vi "NEW_SHIFT_CAL_new.vi"() -> ()   [LabVIEW 2017]
uses:
  <vilib>/addons/database/Connection.llb/DB Tools Open Connec (Path).vi
  <vilib>/addons/database/NI_Database_API.lvlib
panel:
  in  "Cancel Button - Archive":bool
  out "ACTUAL_WORK_TIME":i32
  out "BREAK":i32
  out "LUNCH TIME":i32
  out "In Minutes":i32
  out "error out":errorcluster
  in  "Cycle Time":dbl
  out "x-y":dbl
  out "x-y 8":dbl
  out "x-y 7":dbl
  in  "INCLUDED 9":bool=TRUE
  in  "INCLUDED 8":bool=TRUE
  in  "INCLUDED 7":bool=TRUE
  in  "INCLUDED 6":bool=TRUE
  in  "INCLUDED 5":bool=TRUE
  in  "INCLUDED 4":bool=TRUE
  in  "INCLUDED 3":bool=TRUE
  in  "Include 2":bool=TRUE
  in  "Include":bool=TRUE
  in  "EXTRA SHIFT INCLUDED":bool=TRUE
  in  "Save Button":bool
  in  "Cluster 12":T1 {"1Start 4" format="%<%H:%M:%S>T"; "1Start 3" format="%<%H:%M:%S>T"; "1Start 2" format="%<%H:%M:%S>T"; "1Start" format="%<%H:%M:%S>T"}
  in  "Cluster 11":T1 {"1Start 4" format="%<%H:%M:%S>T"; "1Start 3" format="%<%H:%M:%S>T"; "1Start 2" format="%<%H:%M:%S>T"; "1Start" format="%<%H:%M:%S>T"}
  in  "Cluster 10":T1 {"1Start 4" format="%<%H:%M:%S>T"; "1Start 3" format="%<%H:%M:%S>T"; "1Start 2" format="%<%H:%M:%S>T"; "1Start" format="%<%H:%M:%S>T"}
  in  "Cluster 9":T1 {"1Start 4" format="%<%H:%M:%S>T"; "1Start 3" format="%<%H:%M:%S>T"; "1Start 2" format="%<%H:%M:%S>T"; "1Start" format="%<%H:%M:%S>T"}
  in  "Cluster 8":T2 {"1Start 8" format="%<%H:%M:%S>T"; "1Start 7" format="%<%H:%M:%S>T"; "1Start 6" format="%<%H:%M:%S>T"; "1Start 5" format="%<%H:%M:%S>T"; "1Start 4" format="%<%H:%M:%S>T"; "1Start 3" format="%<%H:%M:%S>T"; "1Start 2" format="%<%H:%M:%S>T"; "1Start" format="%<%H:%M:%S>T"}
  in  "Cluster 7":T2 {"1Start 8" format="%<%H:%M:%S>T"; "1Start 7" format="%<%H:%M:%S>T"; "1Start 6" format="%<%H:%M:%S>T"; "1Start 5" format="%<%H:%M:%S>T"; "1Start 4" format="%<%H:%M:%S>T"; "1Start 3" format="%<%H:%M:%S>T"; "1Start 2" format="%<%H:%M:%S>T"; "1Start" format="%<%H:%M:%S>T"}
  in  "Cluster 6":T2 {"1Start 8" format="%<%H:%M:%S>T"; "1Start 7" format="%<%H:%M:%S>T"; "1Start 6" format="%<%H:%M:%S>T"; "1Start 5" format="%<%H:%M:%S>T"; "1Start 4" format="%<%H:%M:%S>T"; "1Start 3" format="%<%H:%M:%S>T"; "1Start 2" format="%<%H:%M:%S>T"; "1Start" format="%<%H:%M:%S>T"}
  in  "Cluster 5":T2 {"1Start 8" format="%<%H:%M:%S>T"; "1Start 7" format="%<%H:%M:%S>T"; "1Start 6" format="%<%H:%M:%S>T"; "1Start 5" format="%<%H:%M:%S>T"; "1Start 4" format="%<%H:%M:%S>T"; "1Start 3" format="%<%H:%M:%S>T"; "1Start 2" format="%<%H:%M:%S>T"; "1Start" format="%<%H:%M:%S>T"}
  in  "Blank Button":bool
  in  "Cluster 4":T3 {"1Start 6" format="%<%H:%M:%S>T"; "1Start 5" format="%<%H:%M:%S>T"; "1Start 4" format="%<%H:%M:%S>T"; "1Start 3" format="%<%H:%M:%S>T"; "1Start 2" format="%<%H:%M:%S>T"; "1Start" format="%<%H:%M:%S>T"}
  in  "Cluster 3":T3 {"1Start 6" format="%<%I:%M:%S %p>T"; "1Start 5" format="%<%I:%M:%S %p>T"; "1Start 4" format="%<%I:%M:%S %p>T"; "1Start 3" format="%<%I:%M:%S %p>T"; "1Start 2" format="%<%I:%M:%S %p>T"; "1Start" format="%<%I:%M:%S %p>T"}
  in  "Cluster 2":T3 {"1Start 2" format="%<%I:%M:%S %p>T"; "1Start" format="%<%I:%M:%S %p>T"; "1Start 6" format="%<%I:%M:%S %p>T"; "1Start 5" format="%<%I:%M:%S %p>T"; "1Start 4" format="%<%I:%M:%S %p>T"; "1Start 3" format="%<%I:%M:%S %p>T"}
  in  "Cluster":T3 {"1Start 6" format="%<%I:%M:%S %p>T"; "1Start 5" format="%<%I:%M:%S %p>T"; "1Start 4" format="%<%I:%M:%S %p>T"; "1Start 3" format="%<%I:%M:%S %p>T"; "1Start 2" format="%<%I:%M:%S %p>T"; "1Start" format="%<%I:%M:%S %p>T"}
  # "SHIFT SETTING"
  # "06:00:00"
  # "17:59:59"
  # "Sec"
  # "EXTRA SHIFT"
  # "X"
  # "Y"
  # "A"
  # "B"
  # "C"
  # "D"
  # "BREAK 3"
  # "START"
  # "END"
  # "LUNCH"
  # "START"
  # "END"
  # "BREAK 1"
  # "START"
  # "END"
  # "SHIFT IN DAY"
  # "CODE"
  # "START"
  # "END"
  # "A"
  # "B"
  # "C"
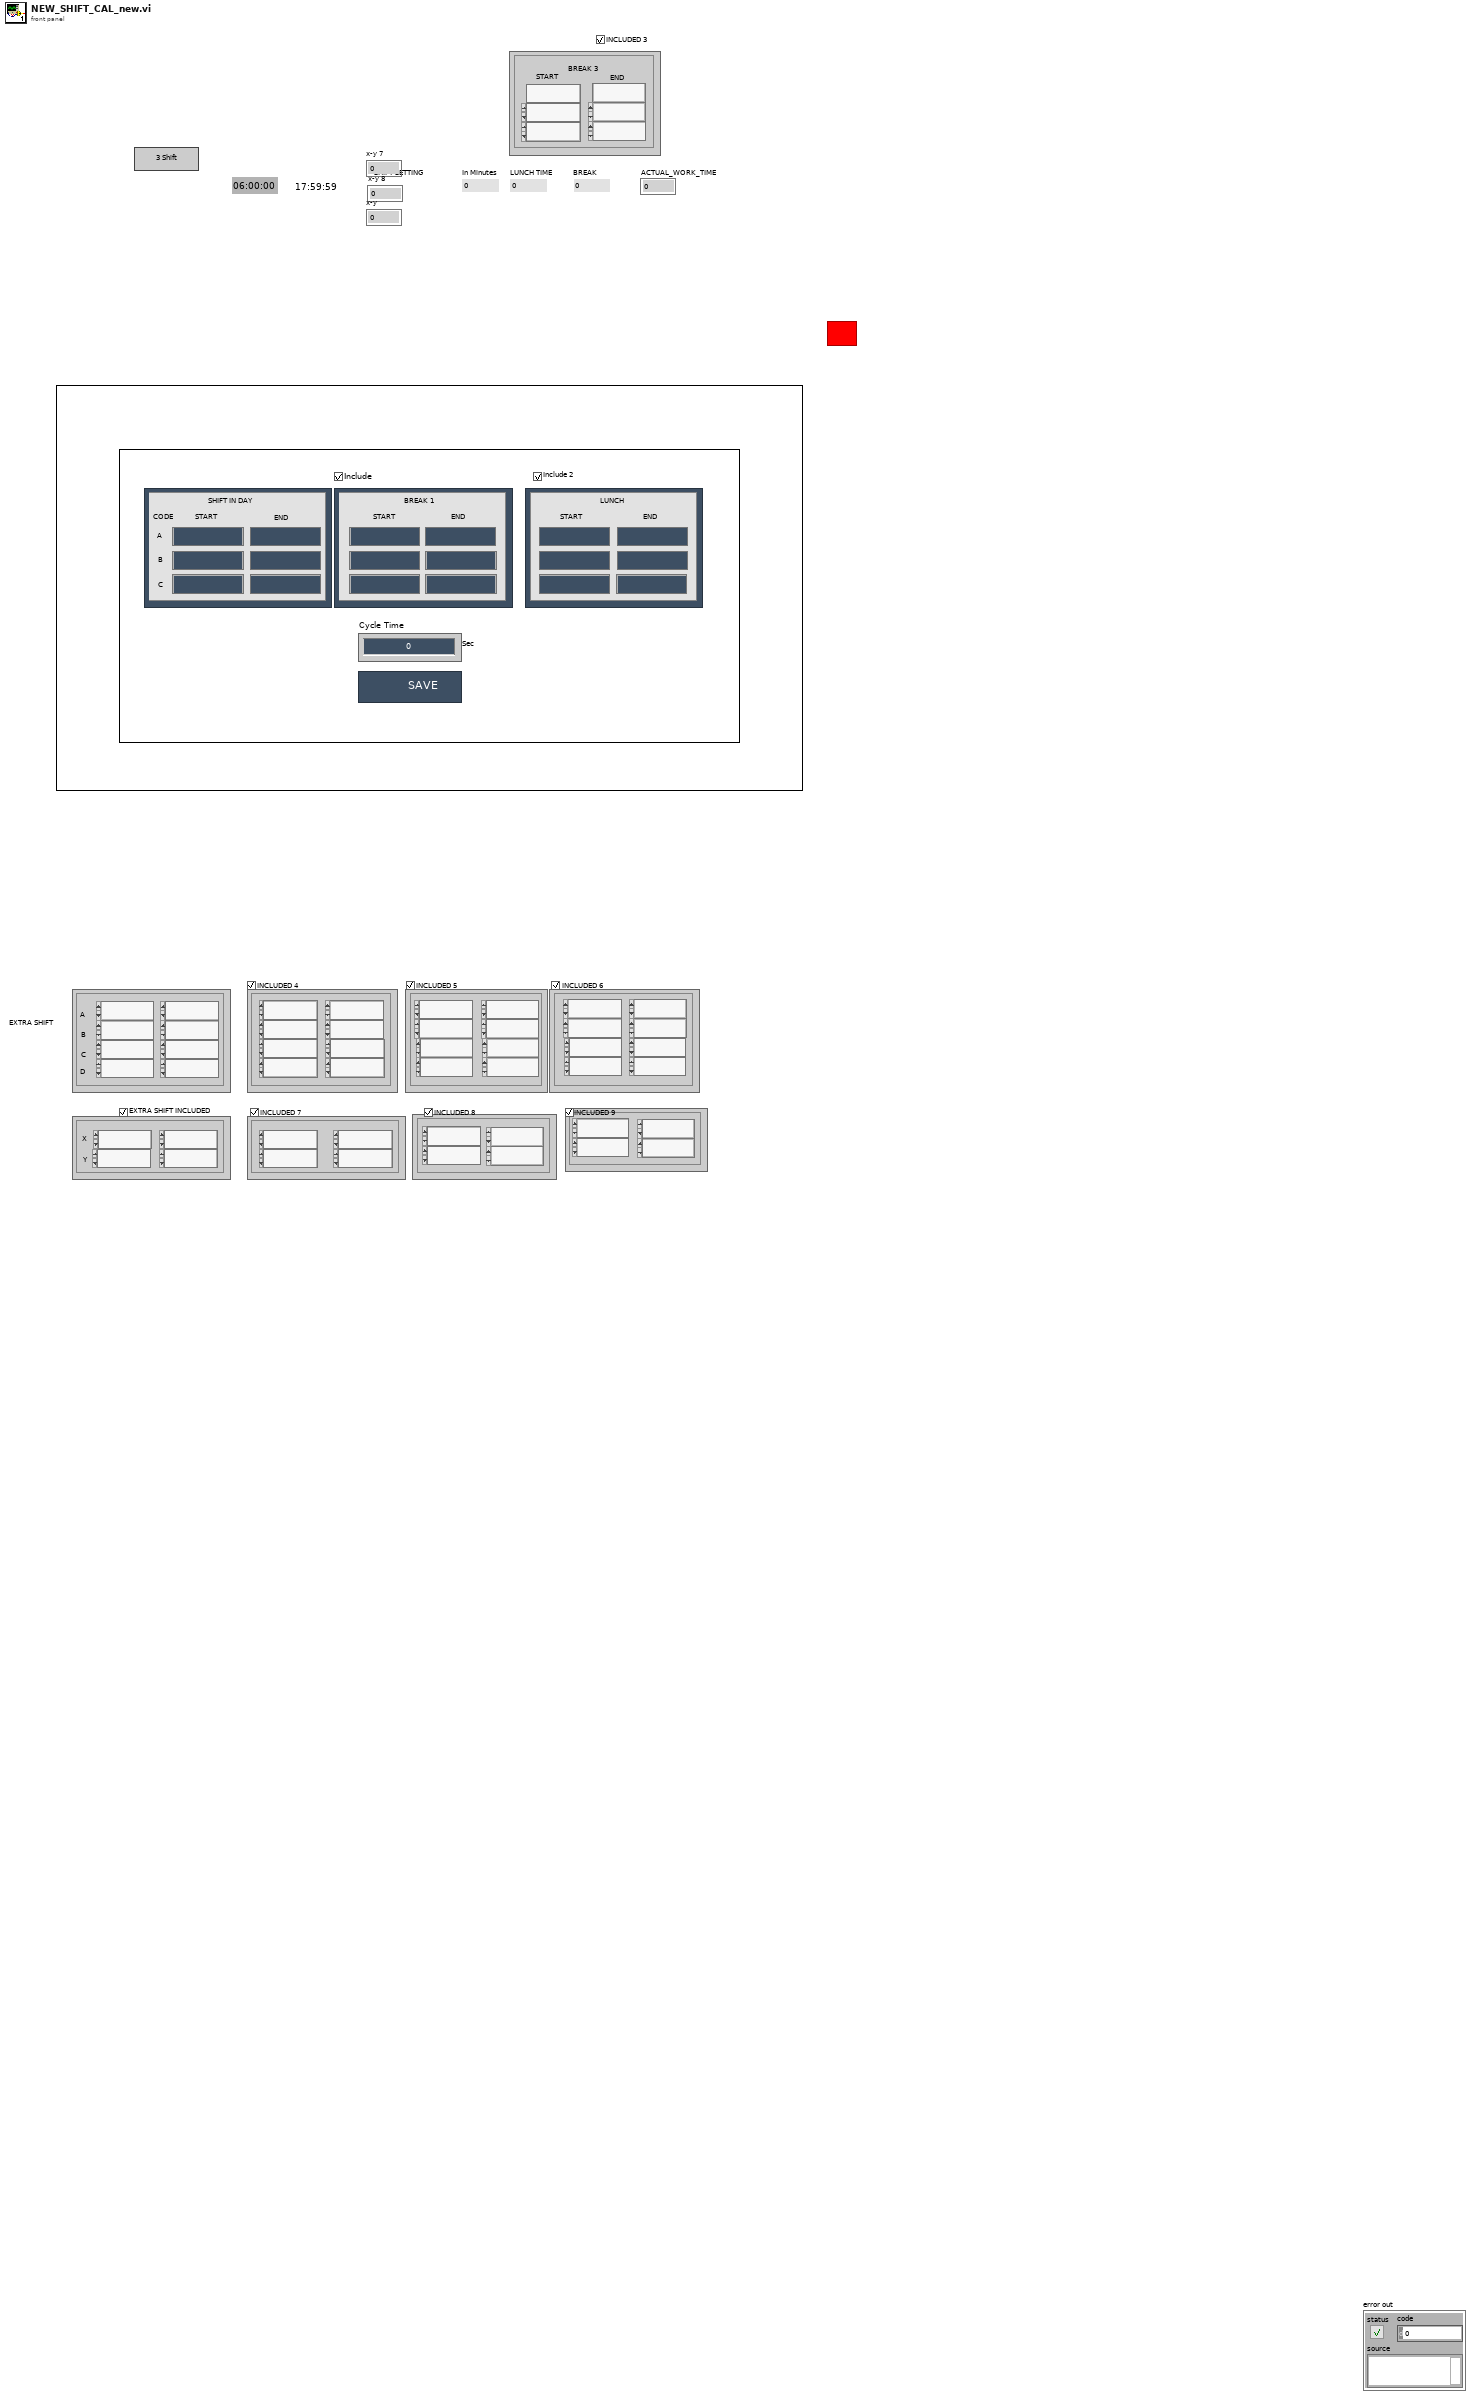
[diagram p1: front panel]
types:
  T1 = cluster{"1Start":timestamp, "1Start 2":timestamp, "1Start 3":timestamp, "1Start 4":timestamp}
  T2 = cluster{"1Start":timestamp, "1Start 2":timestamp, "1Start 3":timestamp, "1Start 4":timestamp, "1Start 5":timestamp, "1Start 6":timestamp, "1Start 7":timestamp, "1Start 8":timestamp}
  T3 = cluster{"1Start":timestamp, "1Start 2":timestamp, "1Start 3":timestamp, "1Start 4":timestamp, "1Start 5":timestamp, "1Start 6":timestamp}
  T4 = typedef "NI_Database_API.lvlib/Conn ObjectReference.ctl" = refnum<k1>
  T5 = cluster{"Time Stamp Out[0]":timestamp, "Time Stamp Out[1]":timestamp, "Time Stamp Out[2]":timestamp, "Time Stamp Out[3]":timestamp}
  T6 = cluster{"Time Stamp Out[0]":timestamp, "Time Stamp Out[1]":timestamp, "Time Stamp Out[2]":timestamp, "Time Stamp Out[3]":timestamp, "Time Stamp Out[4]":timestamp, "Time Stamp Out[5]":timestamp}
  T7 = cluster{"Time Stamp Out[0]":timestamp, "Time Stamp Out[1]":timestamp, "Time Stamp Out[2]":timestamp, "Time Stamp Out[3]":timestamp, "Time Stamp Out[4]":timestamp, "Time Stamp Out[5]":timestamp, "Time Stamp Out[6]":timestamp, "Time Stamp Out[7]":timestamp}
  T8 = cluster{"INCLUDED 9":bool, "date/time string":string, "date/time string":string, "date/time string":string, "date/time string":string}
  T9 = cluster{"INCLUDED 7":bool, "date/time string":string, "date/time string":string, "date/time string":string, "date/time string":string}
  T10 = cluster{"EXTRA SHIFT INCLUDED":bool, "date/time string":string, "date/time string":string, "date/time string":string, "date/time string":string}
  T11 = cluster{"INCLUDED 8":bool, "date/time string":string, "date/time string":string, "date/time string":string, "date/time string":string}
  T12 = cluster{"Include":bool, "date/time string":string, "date/time string":string, "date/time string":string, "date/time string":string, "date/time string":string, "date/time string":string, "In Minutes":i32}
  T13 = cluster{"INCLUDED 4":bool, "date/time string":string, "date/time string":string, "date/time string":string, "date/time string":string, "date/time string":string, "date/time string":string, "date/time string":string, "date/time string":string}
  T14 = cluster{"date/time string":string, "date/time string":string, "date/time string":string, "date/time string":string, "date/time string":string, "date/time string":string, "date/time string":string, "date/time string":string}
  T15 = cluster{"INCLUDED 6":bool, "date/time string":string, "date/time string":string, "date/time string":string, "date/time string":string, "date/time string":string, "date/time string":string, "date/time string":string, "date/time string":string}
  T16 = cluster{"INCLUDED 5":bool, "date/time string":string, "date/time string":string, "date/time string":string, "date/time string":string, "date/time string":string, "date/time string":string, "date/time string":string, "date/time string":string}
  T17 = cluster{"Include 2":bool, "date/time string":string, "date/time string":string, "date/time string":string, "date/time string":string, "date/time string":string, "date/time string":string, "In Minutes":i32}
  T18 = cluster{"INCLUDED 3":bool, "date/time string":string, "date/time string":string, "date/time string":string, "date/time string":string, "date/time string":string, "date/time string":string}
  T19 = cluster{"Blank Button":bool, "date/time string":string, "date/time string":string, "date/time string":string, "date/time string":string, "date/time string":string, "date/time string":string, "In Minutes":i32, i32}
  T20 = cluster{"Time":string, "Time":string, "In Minutes":i32}
  T21 = cluster{"Time":string, "Time":string, "In Minutes":i32}[]
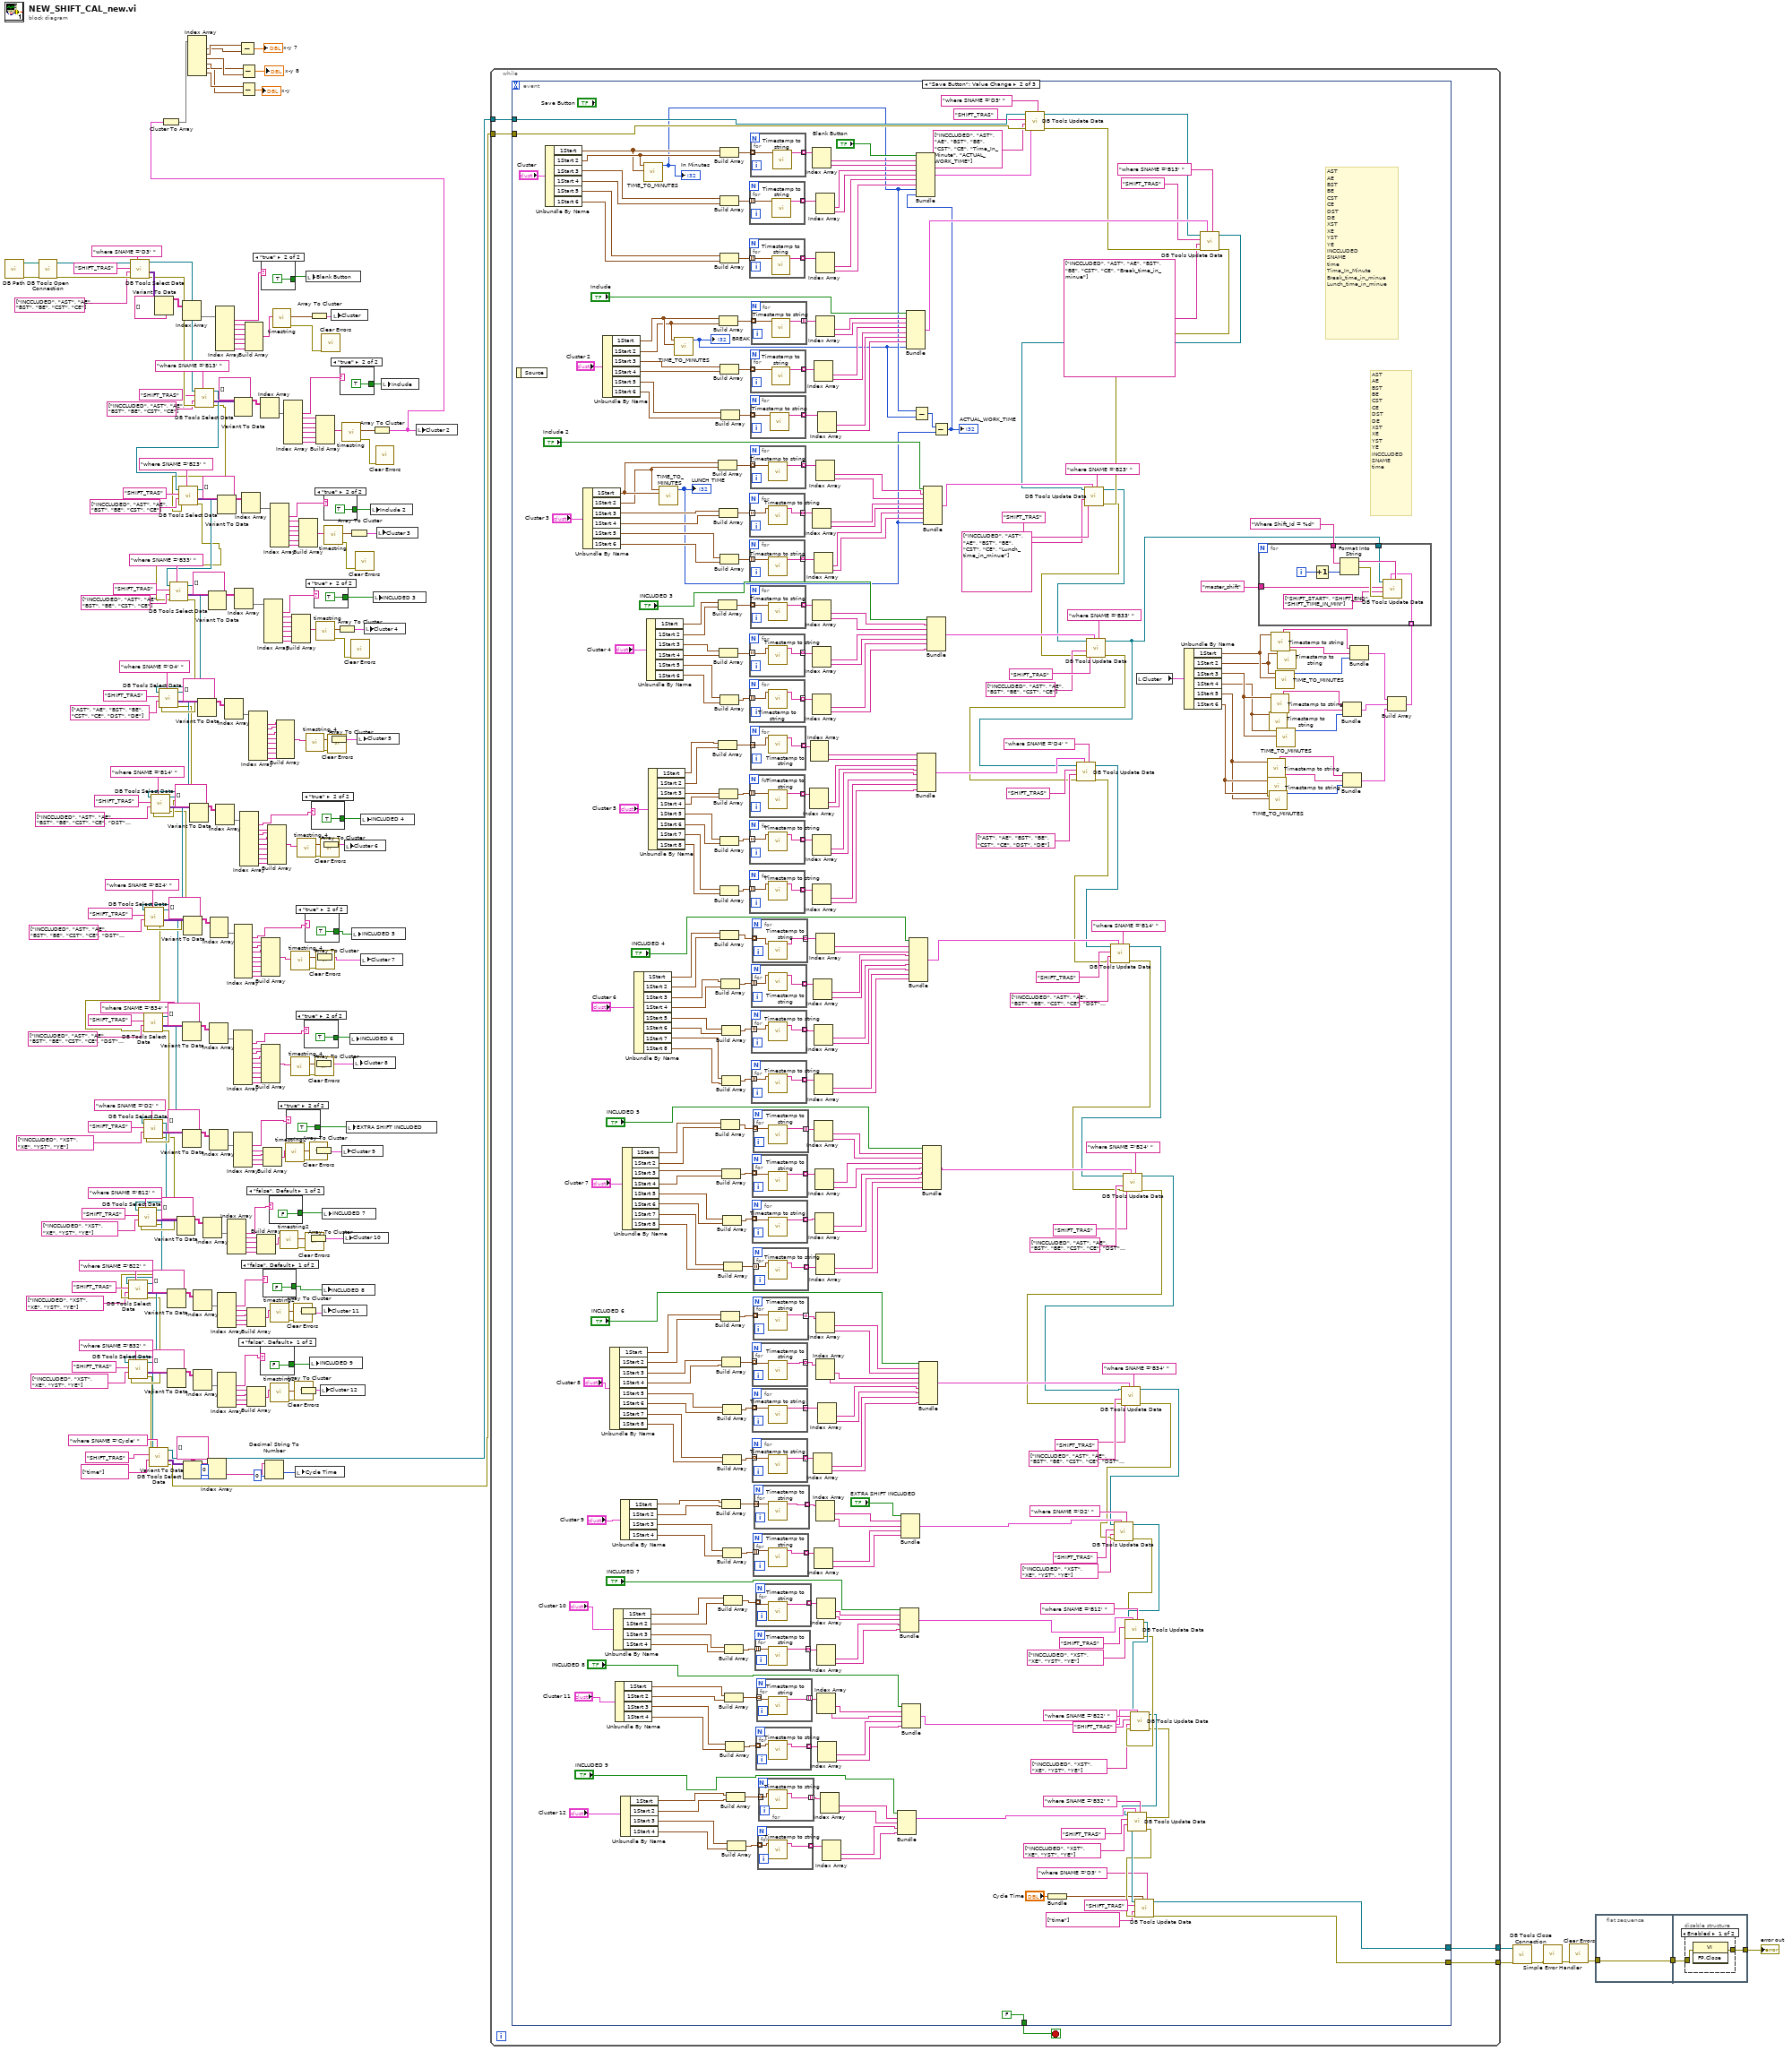
[diagram p0: block diagram]
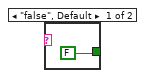
[diagram p3: hidden frame]
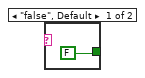
[diagram p4: hidden frame]
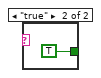
[diagram p5: hidden frame]
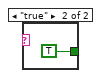
[diagram p6: hidden frame]
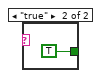
[diagram p7: hidden frame]
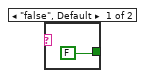
[diagram p8: hidden frame]
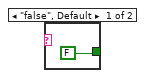
[diagram p9: hidden frame]
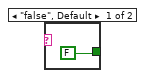
[diagram p10: hidden frame]
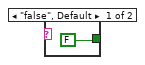
[diagram p11: hidden frame]
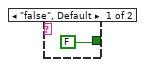
[diagram p12: hidden frame]
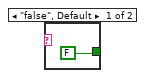
[diagram p13: hidden frame]
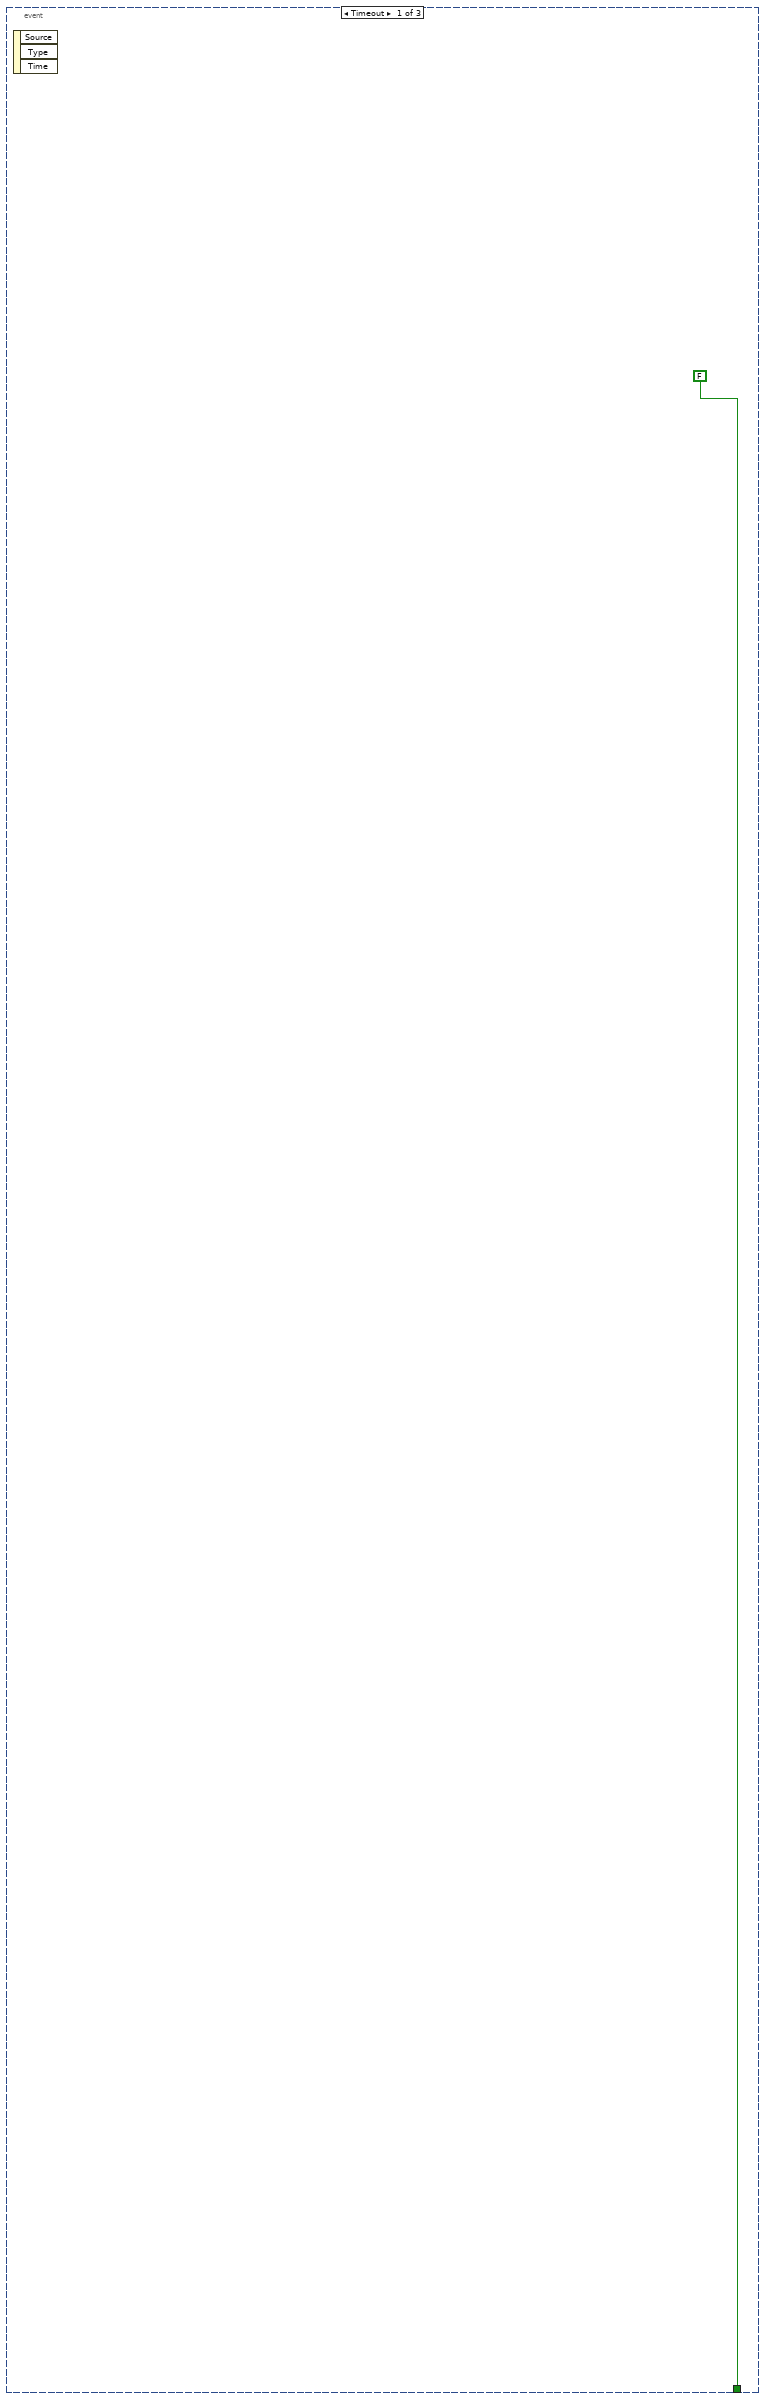
[diagram p14: hidden frame]
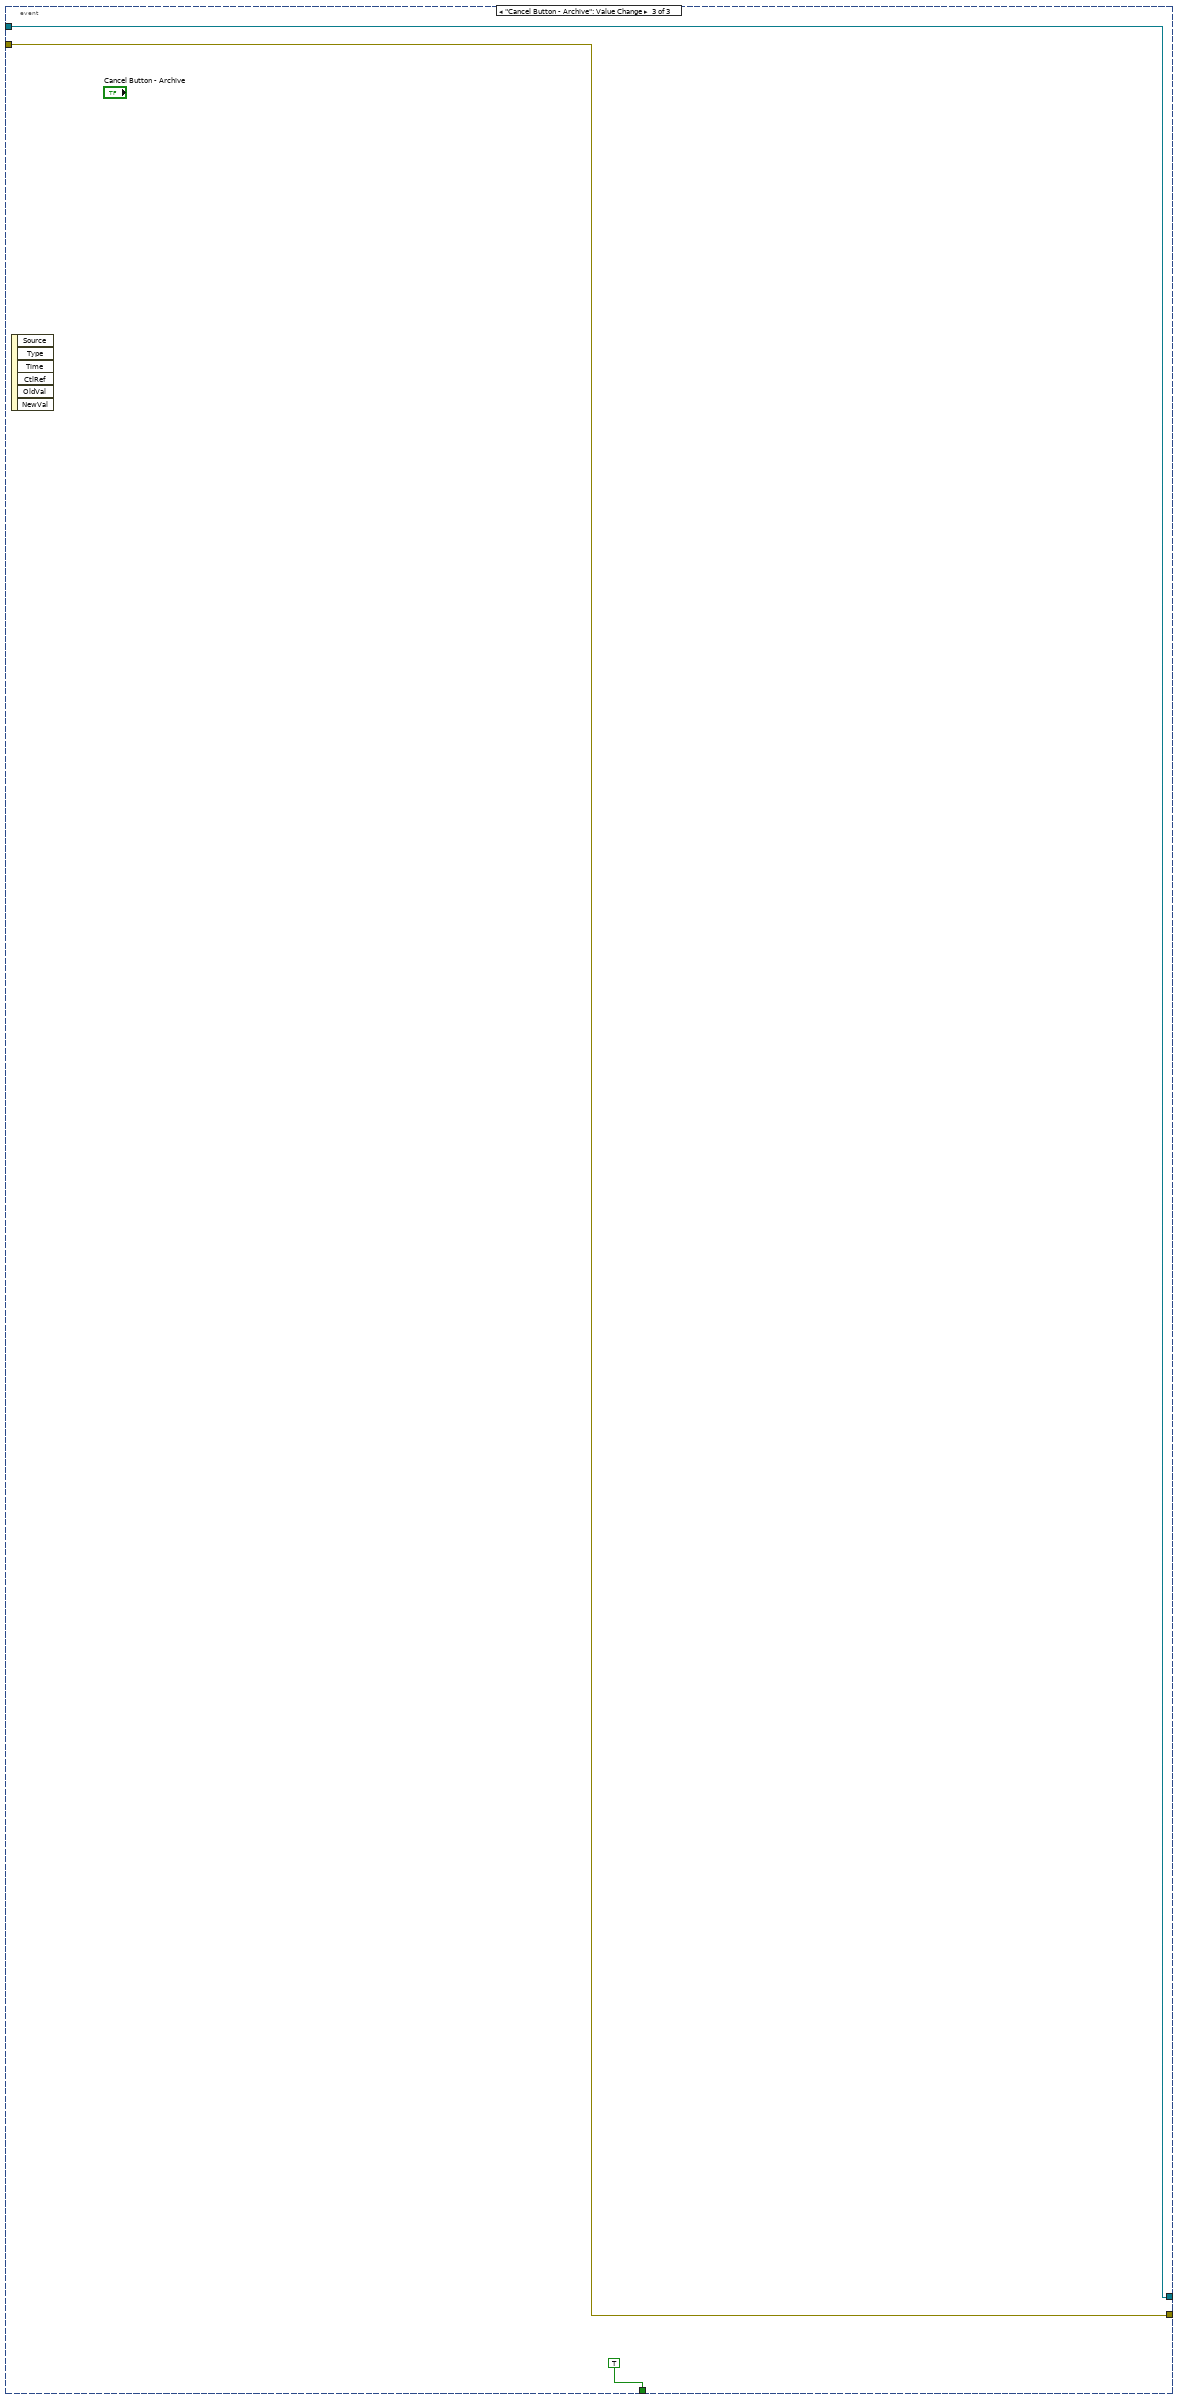
[diagram p15: hidden frame]
diagram:
  n1 = call "DB Path.vi"() -> ("error out"=w283:errorcluster, "DB Path"=w284:path)  [unwired: 10 in]
  n2 = call-poly <vilib>:"DB Tools Open Connection.vi"("error in (no error)"=w283, "connection information"=w284) -> ("error out"=w280:errorcluster, "connection reference"=w279:T4)  [unwired: 6 in]
  n3 = call <vilib>:"DB Tools Select Data.vi"("condition"="where SNAME ='D3' ", "error in (no error)"=w280, "columns"=string[] ["INCCLUDED", "AST", "AE", "BST", "BE", "CST", "CE"], "table"="SHIFT_TRAS", "connection reference"=w279) -> ("error out"=w271:errorcluster, "data"=w276:variant[][], "connection reference out"=w270:T4)  [unwired: 1 in]
  n4 = Variant To Data(type=string[][] [], Variant=w276) -> (data=w274:string[][])  [unwired: 1 in, 1 out]
  n5 = Index Array(array=w274) -> (element=w42:string[])  [unwired: 2 in]
  n6 = call <vilib>:"DB Tools Select Data.vi"("condition"="where SNAME ='B13' ", "error in (no error)"=w271, "columns"=string[] ["INCCLUDED", "AST", "AE", "BST", "BE", "CST", "CE"], "table"="SHIFT_TRAS", "connection reference"=w270) -> ("error out"=w61:errorcluster, "data"=w266:variant[][], "connection reference out"=w216:T4)  [unwired: 1 in]
  n7 = call <vilib>:"DB Tools Select Data.vi"("condition"="where SNAME ='B23' ", "error in (no error)"=w61, "columns"=string[] ["INCCLUDED", "AST", "AE", "BST", "BE", "CST", "CE"], "table"="SHIFT_TRAS", "connection reference"=w216) -> ("error out"=w214:errorcluster, "data"=w240:variant[][], "connection reference out"=w215:T4)  [unwired: 1 in]
  n8 = call <vilib>:"DB Tools Select Data.vi"("condition"="where SNAME ='B33' ", "error in (no error)"=w214, "columns"=string[] ["INCCLUDED", "AST", "AE", "BST", "BE", "CST", "CE"], "table"="SHIFT_TRAS", "connection reference"=w215) -> ("error out"=w194:errorcluster, "data"=w233:variant[][], "connection reference out"=w195:T4)  [unwired: 1 in]
  n9 = call <vilib>:"DB Tools Select Data.vi"("condition"="where SNAME ='D4' ", "error in (no error)"=w194, "columns"=string[] ["AST", "AE", "BST", "BE", "CST", "CE", "DST", "DE"], "table"="SHIFT_TRAS", "connection reference"=w195) -> ("error out"=w74:errorcluster, "data"=w202:variant[][], "connection reference out"=w75:T4)  [unwired: 1 in]
  n10 = call <vilib>:"DB Tools Select Data.vi"("condition"="where SNAME ='B14' ", "error in (no error)"=w74, "columns"=string[] ["INCCLUDED", "AST", "AE", "BST", "BE", "CST", "CE", "DST", "DE"], "table"="SHIFT_TRAS", "connection reference"=w75) -> ("error out"=w72:errorcluster, "data"=w189:variant[][], "connection reference out"=w73:T4)  [unwired: 1 in]
  n11 = call <vilib>:"DB Tools Select Data.vi"("condition"="where SNAME ='B24' ", "error in (no error)"=w72, "columns"=string[] ["INCCLUDED", "AST", "AE", "BST", "BE", "CST", "CE", "DST", "DE"], "table"="SHIFT_TRAS", "connection reference"=w73) -> ("error out"=w70:errorcluster, "data"=w160:variant[][], "connection reference out"=w71:T4)  [unwired: 1 in]
  n12 = call <vilib>:"DB Tools Select Data.vi"("condition"="where SNAME ='B34' ", "error in (no error)"=w70, "columns"=string[] ["INCCLUDED", "AST", "AE", "BST", "BE", "CST", "CE", "DST", "DE"], "table"="SHIFT_TRAS", "connection reference"=w71) -> ("error out"=w68:errorcluster, "data"=w151:variant[][], "connection reference out"=w69:T4)  [unwired: 1 in]
  n13 = call <vilib>:"DB Tools Select Data.vi"("condition"="where SNAME ='D2' ", "error in (no error)"=w68, "columns"=string[] ["INCCLUDED", "XST", "XE", "YST", "YE"], "table"="SHIFT_TRAS", "connection reference"=w69) -> ("error out"=w66:errorcluster, "data"=w128:variant[][], "connection reference out"=w67:T4)  [unwired: 1 in]
  n14 = call <vilib>:"DB Tools Select Data.vi"("condition"="where SNAME ='B12' ", "error in (no error)"=w66, "columns"=string[] ["INCCLUDED", "XST", "XE", "YST", "YE"], "table"="SHIFT_TRAS", "connection reference"=w67) -> ("error out"=w64:errorcluster, "data"=w114:variant[][], "connection reference out"=w65:T4)  [unwired: 1 in]
  n15 = call <vilib>:"DB Tools Select Data.vi"("condition"="where SNAME ='B22' ", "error in (no error)"=w64, "columns"=string[] ["INCCLUDED", "XST", "XE", "YST", "YE"], "table"="SHIFT_TRAS", "connection reference"=w65) -> ("error out"=w62:errorcluster, "data"=w103:variant[][], "connection reference out"=w63:T4)  [unwired: 1 in]
  n16 = call <vilib>:"DB Tools Select Data.vi"("condition"="where SNAME ='B32' ", "error in (no error)"=w62, "columns"=string[] ["INCCLUDED", "XST", "XE", "YST", "YE"], "table"="SHIFT_TRAS", "connection reference"=w63) -> ("error out"=w13:errorcluster, "data"=w90:variant[][], "connection reference out"=w14:T4)  [unwired: 1 in]
  n17 = call <vilib>:"DB Tools Select Data.vi"("condition"="where SNAME ='Cycle' ", "error in (no error)"=w13, "columns"=string[] ["time"], "table"="SHIFT_TRAS", "connection reference"=w14) -> ("error out"=w12:errorcluster, "data"=w18:variant[][], "connection reference out"=w11:T4)  [unwired: 1 in]
  n18 = Variant To Data(type=string[][] [], Variant=w103) -> (data=w105:string[][])  [unwired: 1 in, 1 out]
  n19 = Variant To Data(type=string[][] [], Variant=w90) -> (data=w88:string[][])  [unwired: 1 in, 1 out]
  n20 = Variant To Data(type=string[][] [], Variant=w114) -> (data=w112:string[][])  [unwired: 1 in, 1 out]
  n21 = Variant To Data(type=string[][] [], Variant=w151) -> (data=w149:string[][])  [unwired: 1 in, 1 out]
  n22 = Variant To Data(type=string[][] [], Variant=w128) -> (data=w130:string[][])  [unwired: 1 in, 1 out]
  n23 = Variant To Data(type=string[][] [], Variant=w160) -> (data=w162:string[][])  [unwired: 1 in, 1 out]
  n24 = Variant To Data(type=string[][] [], Variant=w18) -> (data=w16:string[][])  [unwired: 1 in, 1 out]
  n25 = Variant To Data(type=string[][] [], Variant=w189) -> (data=w187:string[][])  [unwired: 1 in, 1 out]
  n26 = Index Array(array=w105) -> (element=w106:string[])  [unwired: 2 in]
  n27 = Index Array(array=w88) -> (element=w87:string[])  [unwired: 2 in]
  n28 = Variant To Data(type=string[][] [], Variant=w202) -> (data=w204:string[][])  [unwired: 1 in, 1 out]
  n29 = Index Array(array=w112) -> (element=w111:string[])  [unwired: 2 in]
  n30 = Index Array(array=w16, index (row)=0, index (col)=0 ("disabled index (col)")) -> (element=w8:string)
  n31 = Variant To Data(type=string[][] [], Variant=w233) -> (data=w231:string[][])  [unwired: 1 in, 1 out]
  n32 = Index Array(array=w149) -> (element=w148:string[])  [unwired: 2 in]
  n33 = Index Array(array=w130) -> (element=w131:string[])  [unwired: 2 in]
  n34 = Index Array(array=w162) -> (element=w163:string[])  [unwired: 2 in]
  n35 = Index Array(array=w42) -> (element #1=w34:string, element #2=w40:string, element #3=w39:string, element #4=w38:string, element #5=w37:string, element #6=w36:string, element #7=w35:string)  [unwired: 7 in]
  n36 = Index Array(array=w187) -> (element=w186:string[])  [unwired: 2 in]
  n37 = Variant To Data(type=string[][] [], Variant=w240) -> (data=w242:string[][])  [unwired: 1 in, 1 out]
  n38 = Index Array(array=w106) -> (element #1=w83:string, element #2=w99:string, element #3=w100:string, element #4=w98:string, element #5=w97:string)  [unwired: 5 in]
  n39 = Index Array(array=w87) -> (element #1=w82:string, element #2=w94:string, element #3=w93:string, element #4=w95:string, element #5=w96:string)  [unwired: 5 in]
  n40 = Index Array(array=w204) -> (element=w205:string[])  [unwired: 2 in]
  n41 = Index Array(array=w111) -> (element #1=w84:string, element #2=w118:string, element #3=w117:string, element #4=w119:string, element #5=w120:string)  [unwired: 5 in]
  n42 = Index Array(array=w148) -> (element #1=w138:string, element #2=w155:string, element #3=w147:string, element #4=w146:string, element #5=w145:string, element #6=w144:string, element #7=w143:string, element #8=w142:string, element #9=w154:string)  [unwired: 9 in]
  n43 = Index Array(array=w131) -> (element #1=w44:string, element #2=w124:string, element #3=w125:string, element #4=w122:string, element #5=w121:string)  [unwired: 5 in]
  n44 = Variant To Data(type=string[][] [], Variant=w266) -> (data=w264:string[][])  [unwired: 1 in, 1 out]
  n45 = Index Array(array=w163) -> (element #1=w173:string, element #2=w156:string, element #3=w164:string, element #4=w165:string, element #5=w166:string, element #6=w167:string, element #7=w168:string, element #8=w169:string, element #9=w157:string)  [unwired: 9 in]
  n46 = Index Array(array=w231) -> (element=w230:string[])  [unwired: 2 in]
  n47 = Index Array(array=w186) -> (element #1=w175:string, element #2=w193:string, element #3=w185:string, element #4=w184:string, element #5=w183:string, element #6=w182:string, element #7=w181:string, element #8=w180:string, element #9=w192:string)  [unwired: 9 in]
  n48 = Index Array(array=w242) -> (element=w243:string[])  [unwired: 2 in]
  n49 = Build Array(w40, w39, w38, w37, w36, w35) -> (w41:string[])
  n50 = Build Array(w99, w100, w98, w97) -> (w107:string[])
  n51 = Build Array(w94, w93, w95, w96) -> (w86:string[])
  n52 = Index Array(array=w205) -> (element #1=w197:string, element #2=w206:string, element #3=w207:string, element #4=w208:string, element #5=w209:string, element #6=w210:string, element #7=w211:string, element #8=w198:string)  [unwired: 8 in]
  n53 = Build Array(w118, w117, w119, w120) -> (w110:string[])
  n54 = Index Array(array=w264) -> (element=w263:string[])  [unwired: 2 in]
  n55 = case shown="\"false\", Default" w82 {
    tunnel: [FALSE TRUE] -> w77
    frame "false", Default {
    }
    frame "true" {
    }
  }
  n56 = Build Array(w155, w147, w146, w145, w144, w143, w142, w154) -> (w141:string[])
  n57 = case shown="\"true\"" w34 {
    tunnel: [FALSE TRUE] -> w33
    frame "false", Default {
    }
    frame "true" {
    }
  }
  n58 = Build Array(w156, w164, w165, w166, w167, w168, w169, w157) -> (w170:string[])
  n59 = Build Array(w124, w125, w122, w121) -> (w132:string[])
  n60 = case shown="\"false\", Default" w83 {
    tunnel: [FALSE TRUE] -> w79
    frame "false", Default {
    }
    frame "true" {
    }
  }
  n61 = Index Array(array=w230) -> (element #1=w221:string, element #2=w229:string, element #3=w228:string, element #4=w227:string, element #5=w226:string, element #6=w225:string, element #7=w224:string)  [unwired: 7 in]
  n62 = Decimal String To Number(string=w8, offset=0) -> (number=w7:i32)  [unwired: 1 in, 1 out]
  n63 = Build Array(w193, w185, w184, w183, w182, w181, w180, w192) -> (w179:string[])
  n64 = case shown="\"false\", Default" w84 {
    tunnel: [FALSE TRUE] -> w80
    frame "false", Default {
    }
    frame "true" {
    }
  }
  n65 = Index Array(array=w243) -> (element #1=w252:string, element #2=w244:string, element #3=w245:string, element #4=w246:string, element #5=w247:string, element #6=w248:string, element #7=w249:string)  [unwired: 7 in]
  n66 = call "timestring2.vi"("String Array In"=w107) -> ("error out"=w56:errorcluster, "Time Stamp Out"=w108:timestamp[])  [unwired: 9 in]
  n67 = call "timestring2.vi"("String Array In"=w86) -> ("error out"=w57:errorcluster, "Time Stamp Out"=w85:timestamp[])  [unwired: 9 in]
  n68 = call "timestring.vi"("String Array In"=w41) -> ("error out"=w46:errorcluster, "Time Stamp Out"=w273:timestamp[])  [unwired: 9 in]
  n69 = Build Array(w197, w206, w207, w208, w209, w210, w211, w198) -> (w212:string[])
  n70 = call "timestring2.vi"("String Array In"=w110) -> ("error out"=w55:errorcluster, "Time Stamp Out"=w109:timestamp[])  [unwired: 9 in]
  n71 = Index Array(array=w263) -> (element #1=w254:string, element #2=w262:string, element #3=w261:string, element #4=w260:string, element #5=w259:string, element #6=w258:string, element #7=w257:string)  [unwired: 7 in]
  n72 = call "timestring2.vi"("String Array In"=w132) -> ("error out"=w54:errorcluster, "Time Stamp Out"=w133:timestamp[])  [unwired: 9 in]
  n73 = case shown="\"true\"" w44 {
    tunnel: [FALSE TRUE] -> w43
    frame "false", Default {
    }
    frame "true" {
    }
  }
  n74 = call "timestring_4.vi"("String Array In"=w141) -> ("error out"=w53:errorcluster, "Time Stamp Out"=w140:timestamp[])  [unwired: 9 in]
  n75 = call "timestring_4.vi"("String Array In"=w170) -> ("error out"=w52:errorcluster, "Time Stamp Out"=w171:timestamp[])  [unwired: 9 in]
  n76 = Build Array(w229, w228, w227, w226, w225, w224) -> (w223:string[])
  n77 = call <vilib>:"Clear Errors.vi"("error in (no error)"=w56) -> ()  [unwired: 5 in, 2 out]
  n78 = call <vilib>:"Clear Errors.vi"("error in (no error)"=w57) -> ()  [unwired: 5 in, 2 out]
  n79 = local write "Cycle Time"(w7) -> ()
  n80 = call "timestring_4.vi"("String Array In"=w179) -> ("error out"=w51:errorcluster, "Time Stamp Out"=w178:timestamp[])  [unwired: 9 in]
  n81 = Build Array(w244, w245, w246, w247, w248, w249) -> (w250:string[])
  n82 = Array To Cluster(array=w108) -> (cluster=w78:T5)
  n83 = Array To Cluster(array=w85) -> (cluster=w76:T5)
  n84 = case shown="\"true\"" w138 {
    tunnel: [FALSE TRUE] -> w134
    frame "false", Default {
    }
    frame "true" {
    }
  }
  n85 = case shown="\"true\"" w173 {
    tunnel: [FALSE TRUE] -> w135
    frame "false", Default {
    }
    frame "true" {
    }
  }
  n86 = call <vilib>:"Clear Errors.vi"("error in (no error)"=w55) -> ()  [unwired: 5 in, 2 out]
  n87 = call "timestring_4.vi"("String Array In"=w212) -> ("error out"=w50:errorcluster, "Time Stamp Out"=w213:timestamp[])  [unwired: 9 in]
  n88 = local write "Blank Button"(w33) -> ()
  n89 = Array To Cluster(array=w109) -> (cluster=w81:T5)
  n90 = call <vilib>:"Clear Errors.vi"("error in (no error)"=w54) -> ()  [unwired: 5 in, 2 out]
  n91 = Array To Cluster(array=w273) -> (cluster=w272:T6)
  n92 = local write "INCLUDED 9"(w77) -> ()
  n93 = case shown="\"true\"" w175 {
    tunnel: [FALSE TRUE] -> w174
    frame "false", Default {
    }
    frame "true" {
    }
  }
  n94 = case shown="\"true\"" w221 {
    tunnel: [FALSE TRUE] -> w218
    frame "false", Default {
    }
    frame "true" {
    }
  }
  n95 = Array To Cluster(array=w140) -> (cluster=w136:T7)
  n96 = call <vilib>:"Clear Errors.vi"("error in (no error)"=w53) -> ()  [unwired: 5 in, 2 out]
  n97 = Array To Cluster(array=w133) -> (cluster=w123:T5)
  n98 = Array To Cluster(array=w171) -> (cluster=w137:T7)
  n99 = Build Array(w262, w261, w260, w259, w258, w257) -> (w256:string[])
  n100 = call "timestring.vi"("String Array In"=w223) -> ("error out"=w49:errorcluster, "Time Stamp Out"=w222:timestamp[])  [unwired: 9 in]
  n101 = call <vilib>:"Clear Errors.vi"("error in (no error)"=w52) -> ()  [unwired: 5 in, 2 out]
  n102 = local write "Cluster 12"(w76) -> ()
  n103 = call <vilib>:"Clear Errors.vi"("error in (no error)"=w51) -> ()  [unwired: 5 in, 2 out]
  n104 = call <vilib>:"Clear Errors.vi"("error in (no error)"=w46) -> ()  [unwired: 5 in, 2 out]
  n105 = Array To Cluster(array=w178) -> (cluster=w177:T7)
  n106 = local write "INCLUDED 8"(w79) -> ()
  n107 = local write "Cluster 11"(w78) -> ()
  n108 = local write "INCLUDED 7"(w80) -> ()
  n109 = case shown="\"true\"" w252 {
    tunnel: [FALSE TRUE] -> w220
    frame "false", Default {
    }
    frame "true" {
    }
  }
  n110 = call "timestring.vi"("String Array In"=w250) -> ("error out"=w48:errorcluster, "Time Stamp Out"=w251:timestamp[])  [unwired: 9 in]
  n111 = call <vilib>:"Clear Errors.vi"("error in (no error)"=w50) -> ()  [unwired: 5 in, 2 out]
  n112 = Array To Cluster(array=w213) -> (cluster=w196:T7)
  n113 = local write "Cluster"(w272) -> ()
  n114 = Array To Cluster(array=w222) -> (cluster=w217:T6)
  n115 = case shown="\"true\"" w254 {
    tunnel: [FALSE TRUE] -> w253
    frame "false", Default {
    }
    frame "true" {
    }
  }
  n116 = call "timestring.vi"("String Array In"=w256) -> ("error out"=w47:errorcluster, "Time Stamp Out"=w255:timestamp[])  [unwired: 9 in]
  n117 = local write "Cluster 9"(w123) -> ()
  n118 = local write "Cluster 10"(w81) -> ()
  n119 = local write "Cluster 6"(w177) -> ()
  n120 = local write "EXTRA SHIFT INCLUDED"(w43) -> ()
  n121 = Array To Cluster(array=w251) -> (cluster=w219:T6)
  n122 = local write "INCLUDED 6"(w134) -> ()
  n123 = call <vilib>:"Clear Errors.vi"("error in (no error)"=w49) -> ()  [unwired: 5 in, 2 out]
  n124 = local write "INCLUDED 5"(w135) -> ()
  n125 = local write "Cluster 8"(w136) -> ()
  n126 = call <vilib>:"Clear Errors.vi"("error in (no error)"=w48) -> ()  [unwired: 5 in, 2 out]
  n127 = local write "Cluster 5"(w196) -> ()
  n128 = local write "INCLUDED 4"(w174) -> ()
  n129 = local write "Cluster 7"(w137) -> ()
  n130 = local write "Cluster 4"(w217) -> ()
  n131 = local write "Include 2"(w220) -> ()
  n132 = Array To Cluster(array=w255) -> (cluster=w31:T6)
  n133 = Cluster To Array(cluster=w31) -> (array=w30:timestamp[])
  n134 = Index Array(array=w30) -> (element #1=w28:timestamp, element #2=w29:timestamp, element #3=w26:timestamp, element #4=w25:timestamp, element #5=w22:timestamp, element #6=w23:timestamp)  [unwired: 6 in]
  n135 = Subtract(x=w29, y=w28) -> (x-y=→"x-y 7":dbl)
  n136 = Subtract(x=w25, y=w26) -> (x-y=→"x-y 8":dbl)
  n137 = Subtract(x=w23, y=w22) -> (x-y=→"x-y":dbl)
  n138 = local write "INCLUDED 3"(w218) -> ()
  n139 = call <vilib>:"Clear Errors.vi"("error in (no error)"=w47) -> ()  [unwired: 5 in, 2 out]
  n140 = local write "Cluster 3"(w219) -> ()
  n141 = local write "Include"(w253) -> ()
  n142 = local write "Cluster 2"(w31) -> ()
  n143 = while {
    tunnel: w11 -> [w310]
    tunnel: w12 -> [w309]
    tunnel: [w308] -> w282
    tunnel: [w307] -> w281
    stop <- w311 stop-if-true
    n144 = event shown="[1] \"Save Button\": Value Change" {
      selector: _ -> [_ _ _]
      dyn-events: _ -> [_ _ _]
      timeout: _ -> [_ _ _]
      tunnel: [FALSE FALSE TRUE] -> w311
      tunnel: w310 -> [_ w480 w743]
      tunnel: w309 -> [_ w479 w742]
      tunnel: [_ w359 w743] -> w308
      tunnel: [_ w358 w742] -> w307
      event Timeout {
        n145 = event-data() -> ()  [unwired: 1 in, 3 out]
      }
      event "Save Button": Value Change {
        # "AST\nAE\nBST\nBE\nCST\nCE\nDST\nDE\nXST\nXE\nYST\nYE\nINCCLUDED\nSNAME\ntime\nTime_In_Minute\nBreak_time_in_minue\nLunch_time_in_minue"
        # "AST\nAE\nBST\nBE\nCST\nCE\nDST\nDE\nXST\nXE\nYST\nYE\nINCCLUDED\nSNAME\ntime"
        n146 = event-data() -> ()  [unwired: 1 in, 1 out]
        n147 = Unbundle By Name("Cluster") -> ("1Start"=w350:timestamp, "1Start 2"=w351:timestamp, "1Start 3"=w349:timestamp, "1Start 4"=w348:timestamp, "1Start 5"=w322:timestamp, "1Start 6"=w321:timestamp)
        n148 = Unbundle By Name("Cluster 3") -> ("1Start"=w345:timestamp, "1Start 2"=w344:timestamp, "1Start 3"=w644:timestamp, "1Start 4"=w643:timestamp, "1Start 5"=w642:timestamp, "1Start 6"=w641:timestamp)
        n149 = Unbundle By Name("Cluster 2") -> ("1Start"=w347:timestamp, "1Start 2"=w346:timestamp, "1Start 3"=w652:timestamp, "1Start 4"=w651:timestamp, "1Start 5"=w650:timestamp, "1Start 6"=w649:timestamp)
        n150 = Unbundle By Name("Cluster 8") -> ("1Start"=w586:timestamp, "1Start 2"=w585:timestamp, "1Start 3"=w584:timestamp, "1Start 4"=w583:timestamp, "1Start 5"=w582:timestamp, "1Start 6"=w581:timestamp, "1Start 7"=w580:timestamp, "1Start 8"=w579:timestamp)
        n151 = Unbundle By Name("Cluster 10") -> ("1Start"=w564:timestamp, "1Start 2"=w563:timestamp, "1Start 3"=w562:timestamp, "1Start 4"=w561:timestamp)
        n152 = Unbundle By Name("Cluster 11") -> ("1Start"=w560:timestamp, "1Start 2"=w559:timestamp, "1Start 3"=w558:timestamp, "1Start 4"=w557:timestamp)
        n153 = Unbundle By Name("Cluster 9") -> ("1Start"=w572:timestamp, "1Start 2"=w571:timestamp, "1Start 3"=w570:timestamp, "1Start 4"=w569:timestamp)
        n154 = Unbundle By Name("Cluster 12") -> ("1Start"=w554:timestamp, "1Start 2"=w553:timestamp, "1Start 3"=w552:timestamp, "1Start 4"=w551:timestamp)
        n155 = Unbundle By Name("Cluster 7") -> ("1Start"=w599:timestamp, "1Start 2"=w598:timestamp, "1Start 3"=w597:timestamp, "1Start 4"=w596:timestamp, "1Start 5"=w595:timestamp, "1Start 6"=w594:timestamp, "1Start 7"=w593:timestamp, "1Start 8"=w592:timestamp)
        n156 = Unbundle By Name("Cluster 6") -> ("1Start"=w612:timestamp, "1Start 2"=w611:timestamp, "1Start 3"=w610:timestamp, "1Start 4"=w609:timestamp, "1Start 5"=w608:timestamp, "1Start 6"=w607:timestamp, "1Start 7"=w606:timestamp, "1Start 8"=w605:timestamp)
        n157 = call "TIME_TO_MINUTES.vi"("START TIME"=w350, "END TIME"=w351) -> ("In Minutes"=w343:i32)  [unwired: 9 in]
        "In Minutes" <- w343
        n158 = Unbundle By Name("Cluster 4") -> ("1Start"=w636:timestamp, "1Start 2"=w635:timestamp, "1Start 3"=w634:timestamp, "1Start 4"=w633:timestamp, "1Start 5"=w632:timestamp, "1Start 6"=w631:timestamp)
        n159 = Unbundle By Name("Cluster 5") -> ("1Start"=w625:timestamp, "1Start 2"=w624:timestamp, "1Start 3"=w623:timestamp, "1Start 4"=w622:timestamp, "1Start 5"=w621:timestamp, "1Start 6"=w620:timestamp, "1Start 7"=w619:timestamp, "1Start 8"=w618:timestamp)
        n160 = call "TIME_TO_MINUTES.vi"("START TIME"=w345, "END TIME"=w344) -> ("In Minutes"=w313:i32)  [unwired: 9 in]
        "LUNCH TIME" <- w313
        n161 = call "TIME_TO_MINUTES.vi"("START TIME"=w347, "END TIME"=w346) -> ("In Minutes"=w314:i32)  [unwired: 9 in]
        "BREAK" <- w314
        n162 = Build Array(w345, w344) -> (w647:timestamp[])
        n163 = Build Array(w636, w635) -> (w637:timestamp[])
        n164 = Build Array(w625, w624) -> (w629:timestamp[])
        n165 = Build Array(w347, w346) -> (w653:timestamp[])
        n166 = Build Array(w644, w643) -> (w646:timestamp[])
        n167 = Build Array(w634, w633) -> (w638:timestamp[])
        n168 = Build Array(w623, w622) -> (w628:timestamp[])
        n169 = Build Array(w652, w651) -> (w654:timestamp[])
        n170 = Build Array(w350, w351) -> (w659:timestamp[])
        n171 = Build Array(w349, w348) -> (w657:timestamp[])
        n172 = Build Array(w322, w321) -> (w656:timestamp[])
        n173 = Build Array(w642, w641) -> (w645:timestamp[])
        n174 = Build Array(w632, w631) -> (w639:timestamp[])
        n175 = Build Array(w621, w620) -> (w627:timestamp[])
        n176 = Build Array(w619, w618) -> (w626:timestamp[])
        n177 = Build Array(w612, w611) -> (w613:timestamp[])
        n178 = Build Array(w650, w649) -> (w655:timestamp[])
        n179 = Build Array(w610, w609) -> (w614:timestamp[])
        n180 = Build Array(w599, w598) -> (w603:timestamp[])
        n181 = Build Array(w586, w585) -> (w587:timestamp[])
        n182 = Build Array(w597, w596) -> (w602:timestamp[])
        n183 = Build Array(w584, w583) -> (w588:timestamp[])
        n184 = Build Array(w608, w607) -> (w615:timestamp[])
        n185 = Build Array(w606, w605) -> (w616:timestamp[])
        n186 = Build Array(w572, w571) -> (w574:timestamp[])
        n187 = Build Array(w595, w594) -> (w601:timestamp[])
        n188 = Build Array(w582, w581) -> (w589:timestamp[])
        n189 = Build Array(w580, w579) -> (w590:timestamp[])
        n190 = Build Array(w570, w569) -> (w573:timestamp[])
        n191 = Build Array(w593, w592) -> (w600:timestamp[])
        n192 = Build Array(w564, w563) -> (w567:timestamp[])
        n193 = Build Array(w562, w561) -> (w568:timestamp[])
        n194 = Build Array(w560, w559) -> (w566:timestamp[])
        n195 = Build Array(w558, w557) -> (w565:timestamp[])
        n196 = Build Array(w554, w553) -> (w555:timestamp[])
        n197 = Build Array(w552, w551) -> (w556:timestamp[])
        n198 = for {
          tunnel: w657 -> [w739] mode=indexing
          tunnel: [w738] -> w549 mode=indexing
          n199 = call "Timestamp to string.vi"("time stamp"=w739) -> ("date/time string"=w738:string)  [unwired: 8 in, 2 out]
        }
        n200 = for {
          tunnel: w656 -> [w737] mode=indexing
          tunnel: [w736] -> w548 mode=indexing
          n201 = call "Timestamp to string.vi"("time stamp"=w737) -> ("date/time string"=w736:string)  [unwired: 8 in, 2 out]
        }
        n202 = for {
          tunnel: w646 -> [w727] mode=indexing
          tunnel: [w726] -> w544 mode=indexing
          n203 = call "Timestamp to string.vi"("time stamp"=w727) -> ("date/time string"=w726:string)  [unwired: 8 in, 2 out]
        }
        n204 = for {
          tunnel: w645 -> [w725] mode=indexing
          tunnel: [w724] -> w542 mode=indexing
          n205 = call "Timestamp to string.vi"("time stamp"=w725) -> ("date/time string"=w724:string)  [unwired: 8 in, 2 out]
        }
        n206 = for {
          tunnel: w638 -> [w721] mode=indexing
          tunnel: [w720] -> w540 mode=indexing
          n207 = call "Timestamp to string.vi"("time stamp"=w721) -> ("date/time string"=w720:string)  [unwired: 8 in, 2 out]
        }
        n208 = for {
          tunnel: w639 -> [w719] mode=indexing
          tunnel: [w718] -> w539 mode=indexing
          n209 = call "Timestamp to string.vi"("time stamp"=w719) -> ("date/time string"=w718:string)  [unwired: 8 in, 2 out]
        }
        n210 = for {
          tunnel: w628 -> [w715] mode=indexing
          tunnel: [w714] -> w537 mode=indexing
          n211 = call "Timestamp to string.vi"("time stamp"=w715) -> ("date/time string"=w714:string)  [unwired: 8 in, 2 out]
        }
        n212 = for {
          tunnel: w627 -> [w713] mode=indexing
          tunnel: [w712] -> w536 mode=indexing
          n213 = call "Timestamp to string.vi"("time stamp"=w713) -> ("date/time string"=w712:string)  [unwired: 8 in, 2 out]
        }
        n214 = for {
          tunnel: w626 -> [w711] mode=indexing
          tunnel: [w710] -> w535 mode=indexing
          n215 = call "Timestamp to string.vi"("time stamp"=w711) -> ("date/time string"=w710:string)  [unwired: 8 in, 2 out]
        }
        n216 = for {
          tunnel: w659 -> [w741] mode=indexing
          tunnel: [w740] -> w550 mode=indexing
          n217 = call "Timestamp to string.vi"("time stamp"=w741) -> ("date/time string"=w740:string)  [unwired: 8 in, 2 out]
        }
        n218 = for {
          tunnel: w654 -> [w732] mode=indexing
          tunnel: [w733] -> w546 mode=indexing
          n219 = call "Timestamp to string.vi"("time stamp"=w732) -> ("date/time string"=w733:string)  [unwired: 8 in, 2 out]
        }
        n220 = for {
          tunnel: w655 -> [w730] mode=indexing
          tunnel: [w731] -> w543 mode=indexing
          n221 = call "Timestamp to string.vi"("time stamp"=w730) -> ("date/time string"=w731:string)  [unwired: 8 in, 2 out]
        }
        n222 = for {
          tunnel: w647 -> [w729] mode=indexing
          tunnel: [w728] -> w545 mode=indexing
          n223 = call "Timestamp to string.vi"("time stamp"=w729) -> ("date/time string"=w728:string)  [unwired: 8 in, 2 out]
        }
        n224 = for {
          tunnel: w637 -> [w723] mode=indexing
          tunnel: [w722] -> w541 mode=indexing
          n225 = call "Timestamp to string.vi"("time stamp"=w723) -> ("date/time string"=w722:string)  [unwired: 8 in, 2 out]
        }
        n226 = for {
          tunnel: w629 -> [w717] mode=indexing
          tunnel: [w716] -> w538 mode=indexing
          n227 = call "Timestamp to string.vi"("time stamp"=w717) -> ("date/time string"=w716:string)  [unwired: 8 in, 2 out]
        }
        n228 = for {
          tunnel: w653 -> [w735] mode=indexing
          tunnel: [w734] -> w547 mode=indexing
          n229 = call "Timestamp to string.vi"("time stamp"=w735) -> ("date/time string"=w734:string)  [unwired: 8 in, 2 out]
        }
        n230 = for {
          tunnel: w614 -> [w707] mode=indexing
          tunnel: [w706] -> w533 mode=indexing
          n231 = call "Timestamp to string.vi"("time stamp"=w707) -> ("date/time string"=w706:string)  [unwired: 8 in, 2 out]
        }
        n232 = for {
          tunnel: w615 -> [w705] mode=indexing
          tunnel: [w704] -> w532 mode=indexing
          n233 = call "Timestamp to string.vi"("time stamp"=w705) -> ("date/time string"=w704:string)  [unwired: 8 in, 2 out]
        }
        n234 = for {
          tunnel: w616 -> [w703] mode=indexing
          tunnel: [w702] -> w531 mode=indexing
          n235 = call "Timestamp to string.vi"("time stamp"=w703) -> ("date/time string"=w702:string)  [unwired: 8 in, 2 out]
        }
        n236 = for {
          tunnel: w613 -> [w709] mode=indexing
          tunnel: [w708] -> w534 mode=indexing
          n237 = call "Timestamp to string.vi"("time stamp"=w709) -> ("date/time string"=w708:string)  [unwired: 8 in, 2 out]
        }
        n238 = for {
          tunnel: w602 -> [w698] mode=indexing
          tunnel: [w699] -> w529 mode=indexing
          n239 = call "Timestamp to string.vi"("time stamp"=w698) -> ("date/time string"=w699:string)  [unwired: 8 in, 2 out]
        }
        n240 = for {
          tunnel: w601 -> [w697] mode=indexing
          tunnel: [w696] -> w528 mode=indexing
          n241 = call "Timestamp to string.vi"("time stamp"=w697) -> ("date/time string"=w696:string)  [unwired: 8 in, 2 out]
        }
        n242 = for {
          tunnel: w588 -> [w691] mode=indexing
          tunnel: [w690] -> w525 mode=indexing
          n243 = call "Timestamp to string.vi"("time stamp"=w691) -> ("date/time string"=w690:string)  [unwired: 8 in, 2 out]
        }
        n244 = for {
          tunnel: w589 -> [w689] mode=indexing
          tunnel: [w688] -> w524 mode=indexing
          n245 = call "Timestamp to string.vi"("time stamp"=w689) -> ("date/time string"=w688:string)  [unwired: 8 in, 2 out]
        }
        n246 = for {
          tunnel: w590 -> [w687] mode=indexing
          tunnel: [w686] -> w523 mode=indexing
          n247 = call "Timestamp to string.vi"("time stamp"=w687) -> ("date/time string"=w686:string)  [unwired: 8 in, 2 out]
        }
        n248 = for {
          tunnel: w603 -> [w701] mode=indexing
          tunnel: [w700] -> w530 mode=indexing
          n249 = call "Timestamp to string.vi"("time stamp"=w701) -> ("date/time string"=w700:string)  [unwired: 8 in, 2 out]
        }
        n250 = for {
          tunnel: w587 -> [w693] mode=indexing
          tunnel: [w692] -> w526 mode=indexing
          n251 = call "Timestamp to string.vi"("time stamp"=w693) -> ("date/time string"=w692:string)  [unwired: 8 in, 2 out]
        }
        n252 = for {
          tunnel: w600 -> [w695] mode=indexing
          tunnel: [w694] -> w527 mode=indexing
          n253 = call "Timestamp to string.vi"("time stamp"=w695) -> ("date/time string"=w694:string)  [unwired: 8 in, 2 out]
        }
        n254 = for {
          tunnel: w573 -> [w683] mode=indexing
          tunnel: [w682] -> w521 mode=indexing
          n255 = call "Timestamp to string.vi"("time stamp"=w683) -> ("date/time string"=w682:string)  [unwired: 8 in, 2 out]
        }
        n256 = for {
          tunnel: w574 -> [w685] mode=indexing
          tunnel: [w684] -> w522 mode=indexing
          n257 = call "Timestamp to string.vi"("time stamp"=w685) -> ("date/time string"=w684:string)  [unwired: 8 in, 2 out]
        }
        n258 = for {
          tunnel: w568 -> [w679] mode=indexing
          tunnel: [w678] -> w519 mode=indexing
          n259 = call "Timestamp to string.vi"("time stamp"=w679) -> ("date/time string"=w678:string)  [unwired: 8 in, 2 out]
        }
        n260 = for {
          tunnel: w567 -> [w681] mode=indexing
          tunnel: [w680] -> w520 mode=indexing
          n261 = call "Timestamp to string.vi"("time stamp"=w681) -> ("date/time string"=w680:string)  [unwired: 8 in, 2 out]
        }
        n262 = for {
          tunnel: w565 -> [w675] mode=indexing
          tunnel: [w674] -> w517 mode=indexing
          n263 = call "Timestamp to string.vi"("time stamp"=w675) -> ("date/time string"=w674:string)  [unwired: 8 in, 2 out]
        }
        n264 = for {
          tunnel: w566 -> [w676] mode=indexing
          tunnel: [w677] -> w518 mode=indexing
          n265 = call "Timestamp to string.vi"("time stamp"=w676) -> ("date/time string"=w677:string)  [unwired: 8 in, 2 out]
        }
        n266 = for {
          tunnel: w556 -> [w671] mode=indexing
          tunnel: [w670] -> w515 mode=indexing
          n267 = call "Timestamp to string.vi"("time stamp"=w671) -> ("date/time string"=w670:string)  [unwired: 8 in, 2 out]
        }
        n268 = for {
          tunnel: w555 -> [w673] mode=indexing
          tunnel: [w672] -> w516 mode=indexing
          n269 = call "Timestamp to string.vi"("time stamp"=w673) -> ("date/time string"=w672:string)  [unwired: 8 in, 2 out]
        }
        n270 = Index Array(array=w537) -> (element #1=w486:string, element #2=w485:string)  [unwired: 2 in]
        n271 = Index Array(array=w538) -> (element #1=w488:string, element #2=w487:string)  [unwired: 2 in]
        n272 = Index Array(array=w544) -> (element #1=w498:string, element #2=w497:string)  [unwired: 2 in]
        n273 = Index Array(array=w541) -> (element #1=w494:string, element #2=w493:string)  [unwired: 2 in]
        n274 = Index Array(array=w540) -> (element #1=w492:string, element #2=w491:string)  [unwired: 2 in]
        n275 = Index Array(array=w539) -> (element #1=w490:string, element #2=w489:string)  [unwired: 2 in]
        n276 = Index Array(array=w535) -> (element #1=w482:string, element #2=w481:string)  [unwired: 2 in]
        n277 = Index Array(array=w550) -> (element #1=w514:string, element #2=w513:string)  [unwired: 2 in]
        n278 = Index Array(array=w536) -> (element #1=w484:string, element #2=w483:string)  [unwired: 2 in]
        n279 = Index Array(array=w533) -> (element #1=w451:string, element #2=w450:string)  [unwired: 2 in]
        n280 = Index Array(array=w523) -> (element #1=w428:string, element #2=w427:string)  [unwired: 2 in]
        n281 = Index Array(array=w542) -> (element #1=w496:string, element #2=w495:string)  [unwired: 2 in]
        n282 = Index Array(array=w532) -> (element #1=w449:string, element #2=w448:string)  [unwired: 2 in]
        n283 = Index Array(array=w530) -> (element #1=w444:string, element #2=w443:string)  [unwired: 2 in]
        n284 = Index Array(array=w546) -> (element #1=w504:string, element #2=w503:string)  [unwired: 2 in]
        n285 = Index Array(array=w531) -> (element #1=w447:string, element #2=w446:string)  [unwired: 2 in]
        n286 = Index Array(array=w521) -> (element #1=w422:string, element #2=w421:string)  [unwired: 2 in]
        n287 = Index Array(array=w529) -> (element #1=w442:string, element #2=w441:string)  [unwired: 2 in]
        n288 = Index Array(array=w528) -> (element #1=w440:string, element #2=w439:string)  [unwired: 2 in]
        n289 = Index Array(array=w549) -> (element #1=w512:string, element #2=w511:string)  [unwired: 2 in]
        n290 = Index Array(array=w548) -> (element #1=w510:string, element #2=w509:string)  [unwired: 2 in]
        n291 = Index Array(array=w547) -> (element #1=w506:string, element #2=w505:string)  [unwired: 2 in]
        n292 = Index Array(array=w526) -> (element #1=w434:string, element #2=w433:string)  [unwired: 2 in]
        n293 = Index Array(array=w525) -> (element #1=w432:string, element #2=w431:string)  [unwired: 2 in]
        n294 = Index Array(array=w522) -> (element #1=w424:string, element #2=w423:string)  [unwired: 2 in]
        n295 = Index Array(array=w545) -> (element #1=w500:string, element #2=w499:string)  [unwired: 2 in]
        n296 = Index Array(array=w534) -> (element #1=w453:string, element #2=w452:string)  [unwired: 2 in]
        n297 = Index Array(array=w527) -> (element #1=w438:string, element #2=w437:string)  [unwired: 2 in]
        n298 = Index Array(array=w520) -> (element #1=w420:string, element #2=w419:string)  [unwired: 2 in]
        n299 = Index Array(array=w519) -> (element #1=w418:string, element #2=w417:string)  [unwired: 2 in]
        n300 = Index Array(array=w518) -> (element #1=w416:string, element #2=w415:string)  [unwired: 2 in]
        n301 = Index Array(array=w543) -> (element #1=w502:string, element #2=w501:string)  [unwired: 2 in]
        n302 = Index Array(array=w524) -> (element #1=w430:string, element #2=w429:string)  [unwired: 2 in]
        n303 = Index Array(array=w517) -> (element #1=w414:string, element #2=w413:string)  [unwired: 2 in]
        n304 = Index Array(array=w516) -> (element #1=w412:string, element #2=w411:string)  [unwired: 2 in]
        n305 = Index Array(array=w515) -> (element #1=w410:string, element #2=w409:string)  [unwired: 2 in]
        n306 = Bundle("INCLUDED 9"="INCLUDED 9", "date/time string"=w412, "date/time string"=w411, "date/time string"=w410, "date/time string"=w409) -> (w398:T8)  [unwired: 1 in]
        n307 = Bundle("INCLUDED 7"="INCLUDED 7", "date/time string"=w420, "date/time string"=w419, "date/time string"=w418, "date/time string"=w417) -> (w404:T9)  [unwired: 1 in]
        n308 = Bundle("EXTRA SHIFT INCLUDED"="EXTRA SHIFT INCLUDED", "date/time string"=w424, "date/time string"=w423, "date/time string"=w422, "date/time string"=w421) -> (w408:T10)  [unwired: 1 in]
        n309 = Bundle("INCLUDED 8"="INCLUDED 8", "date/time string"=w416, "date/time string"=w415, "date/time string"=w414, "date/time string"=w413) -> (w401:T11)  [unwired: 1 in]
        n310 = Bundle("Include"="Include", "date/time string"=w506, "date/time string"=w505, "date/time string"=w504, "date/time string"=w503, "date/time string"=w502, "date/time string"=w501, "In Minutes"=w314) -> (w476:T12)  [unwired: 1 in]
        n311 = Bundle("INCLUDED 4"="INCLUDED 4", "date/time string"=w453, "date/time string"=w452, "date/time string"=w451, "date/time string"=w450, "date/time string"=w449, "date/time string"=w448, "date/time string"=w447, "date/time string"=w446) -> (w445:T13)  [unwired: 1 in]
        n312 = Subtract(x=w343, y=w314) -> (x-y=w342:i32)
        n313 = Bundle("date/time string"=w488, "date/time string"=w487, "date/time string"=w486, "date/time string"=w485, "date/time string"=w484, "date/time string"=w483, "date/time string"=w482, "date/time string"=w481) -> (w463:T14)  [unwired: 1 in]
        n314 = Bundle("INCLUDED 6"="INCLUDED 6", "date/time string"=w434, "date/time string"=w433, "date/time string"=w432, "date/time string"=w431, "date/time string"=w430, "date/time string"=w429, "date/time string"=w428, "date/time string"=w427) -> (w435:T15)  [unwired: 1 in]
        n315 = Bundle("INCLUDED 5"="INCLUDED 5", "date/time string"=w444, "date/time string"=w443, "date/time string"=w442, "date/time string"=w441, "date/time string"=w440, "date/time string"=w439, "date/time string"=w438, "date/time string"=w437) -> (w436:T16)  [unwired: 1 in]
        n316 = Bundle("Include 2"="Include 2", "date/time string"=w500, "date/time string"=w499, "date/time string"=w498, "date/time string"=w497, "date/time string"=w496, "date/time string"=w495, "In Minutes"=w313) -> (w473:T17)  [unwired: 1 in]
        n317 = Bundle("INCLUDED 3"="INCLUDED 3", "date/time string"=w494, "date/time string"=w493, "date/time string"=w492, "date/time string"=w491, "date/time string"=w490, "date/time string"=w489) -> (w467:T18)  [unwired: 1 in]
        n318 = Subtract(x=w342, y=w313) -> (x-y=w341:i32)
        "ACTUAL_WORK_TIME" <- w341
        n319 = Bundle("Blank Button"="Blank Button", "date/time string"=w514, "date/time string"=w513, "date/time string"=w512, "date/time string"=w511, "date/time string"=w510, "date/time string"=w509, "In Minutes"=w343, w341) -> (w508:T19)  [unwired: 1 in]
        n320 = call <vilib>:"DB Tools Update Data.vi"("condition"="where SNAME ='D3' ", "data"=w508, "error in (no error)"=w479, "columns"=string[] ["INCCLUDED", "AST", "AE", "BST", "BE", "CST", "CE", "Time_In_Minute", "ACTUAL_WORK_TIME"], "table"="SHIFT_TRAS", "connection reference"=w480) -> ("error out"=w474:errorcluster, "connection reference out"=w475:T4)  [unwired: 4 in]
        n321 = Bundle("Cycle Time"="Cycle Time") -> (w355:cluster{"Cycle Time":dbl})  [unwired: 1 in]
        n322 = local read "Cluster"() -> (w337:T3)
        n323 = Unbundle By Name(w337) -> ("1Start"=w328:timestamp, "1Start 2"=w327:timestamp, "1Start 3"=w326:timestamp, "1Start 4"=w325:timestamp, "1Start 5"=w323:timestamp, "1Start 6"=w324:timestamp)
        n324 = call <vilib>:"DB Tools Update Data.vi"("condition"="where SNAME ='B13' ", "data"=w476, "error in (no error)"=w474, "columns"=string[] ["INCCLUDED", "AST", "AE", "BST", "BE", "CST", "CE", "Break_time_in_minue"], "table"="SHIFT_TRAS", "connection reference"=w475) -> ("error out"=w396:errorcluster, "connection reference out"=w397:T4)  [unwired: 4 in]
        n325 = call <vilib>:"DB Tools Update Data.vi"("condition"="where SNAME ='B23' ", "data"=w473, "error in (no error)"=w396, "columns"=string[] ["INCCLUDED", "AST", "AE", "BST", "BE", "CST", "CE", "Lunch_time_in_minue"], "table"="SHIFT_TRAS", "connection reference"=w397) -> ("error out"=w394:errorcluster, "connection reference out"=w395:T4)  [unwired: 4 in]
        n326 = call <vilib>:"DB Tools Update Data.vi"("condition"="where SNAME ='B33' ", "data"=w467, "error in (no error)"=w394, "columns"=string[] ["INCCLUDED", "AST", "AE", "BST", "BE", "CST", "CE"], "table"="SHIFT_TRAS", "connection reference"=w395) -> ("error out"=w393:errorcluster, "connection reference out"=w329:T4)  [unwired: 4 in]
        n327 = call <vilib>:"DB Tools Update Data.vi"("condition"="where SNAME ='D4' ", "data"=w463, "error in (no error)"=w393, "columns"=string[] ["AST", "AE", "BST", "BE", "CST", "CE", "DST", "DE"], "table"="SHIFT_TRAS", "connection reference"=w329) -> ("error out"=w391:errorcluster, "connection reference out"=w392:T4)  [unwired: 4 in]
        n328 = call <vilib>:"DB Tools Update Data.vi"("condition"="where SNAME ='B14' ", "data"=w445, "error in (no error)"=w391, "columns"=string[] ["INCCLUDED", "AST", "AE", "BST", "BE", "CST", "CE", "DST", "DE"], "table"="SHIFT_TRAS", "connection reference"=w392) -> ("error out"=w389:errorcluster, "connection reference out"=w390:T4)  [unwired: 4 in]
        n329 = call <vilib>:"DB Tools Update Data.vi"("condition"="where SNAME ='B24' ", "data"=w436, "error in (no error)"=w389, "columns"=string[] ["INCCLUDED", "AST", "AE", "BST", "BE", "CST", "CE", "DST", "DE"], "table"="SHIFT_TRAS", "connection reference"=w390) -> ("error out"=w387:errorcluster, "connection reference out"=w388:T4)  [unwired: 4 in]
        n330 = call <vilib>:"DB Tools Update Data.vi"("condition"="where SNAME ='B34' ", "data"=w435, "error in (no error)"=w387, "columns"=string[] ["INCCLUDED", "AST", "AE", "BST", "BE", "CST", "CE", "DST", "DE"], "table"="SHIFT_TRAS", "connection reference"=w388) -> ("error out"=w385:errorcluster, "connection reference out"=w386:T4)  [unwired: 4 in]
        n331 = call <vilib>:"DB Tools Update Data.vi"("condition"="where SNAME ='D2' ", "data"=w408, "error in (no error)"=w385, "columns"=string[] ["INCCLUDED", "XST", "XE", "YST", "YE"], "table"="SHIFT_TRAS", "connection reference"=w386) -> ("error out"=w383:errorcluster, "connection reference out"=w384:T4)  [unwired: 4 in]
        n332 = call <vilib>:"DB Tools Update Data.vi"("condition"="where SNAME ='B12' ", "data"=w404, "error in (no error)"=w383, "columns"=string[] ["INCCLUDED", "XST", "XE", "YST", "YE"], "table"="SHIFT_TRAS", "connection reference"=w384) -> ("error out"=w381:errorcluster, "connection reference out"=w382:T4)  [unwired: 4 in]
        n333 = call <vilib>:"DB Tools Update Data.vi"("condition"="where SNAME ='B22' ", "data"=w401, "error in (no error)"=w381, "columns"=string[] ["INCCLUDED", "XST", "XE", "YST", "YE"], "table"="SHIFT_TRAS", "connection reference"=w382) -> ("error out"=w379:errorcluster, "connection reference out"=w380:T4)  [unwired: 4 in]
        n334 = call <vilib>:"DB Tools Update Data.vi"("condition"="where SNAME ='B32' ", "data"=w398, "error in (no error)"=w379, "columns"=string[] ["INCCLUDED", "XST", "XE", "YST", "YE"], "table"="SHIFT_TRAS", "connection reference"=w380) -> ("error out"=w360:errorcluster, "connection reference out"=w361:T4)  [unwired: 4 in]
        n335 = call <vilib>:"DB Tools Update Data.vi"("condition"="where SNAME ='D3' ", "data"=w355, "error in (no error)"=w360, "columns"=string[] ["time"], "table"="SHIFT_TRAS", "connection reference"=w361) -> ("error out"=w358:errorcluster, "connection reference out"=w359:T4)  [unwired: 4 in]
        n336 = call "Timestamp to string.vi"("time stamp"=w323) -> ("Time"=w316:string)  [unwired: 8 in, 2 out]
        n337 = call "Timestamp to string.vi"("time stamp"=w324) -> ("Time"=w315:string)  [unwired: 8 in, 2 out]
        n338 = call "Timestamp to string.vi"("time stamp"=w325) -> ("Time"=w317:string)  [unwired: 8 in, 2 out]
        n339 = call "TIME_TO_MINUTES.vi"("START TIME"=w323, "END TIME"=w324) -> ("In Minutes"=w330:i32)  [unwired: 9 in]
        n340 = call "Timestamp to string.vi"("time stamp"=w326) -> ("Time"=w318:string)  [unwired: 8 in, 2 out]
        n341 = call "Timestamp to string.vi"("time stamp"=w328) -> ("Time"=w320:string)  [unwired: 8 in, 2 out]
        n342 = call "TIME_TO_MINUTES.vi"("START TIME"=w328, "END TIME"=w327) -> ("In Minutes"=w332:i32)  [unwired: 9 in]
        n343 = call "TIME_TO_MINUTES.vi"("START TIME"=w326, "END TIME"=w325) -> ("In Minutes"=w331:i32)  [unwired: 9 in]
        n344 = call "Timestamp to string.vi"("time stamp"=w327) -> ("Time"=w319:string)  [unwired: 8 in, 2 out]
        n345 = Bundle("Time"=w318, "Time"=w317, "In Minutes"=w331) -> (w335:T20)  [unwired: 1 in]
        n346 = Bundle("Time"=w316, "Time"=w315, "In Minutes"=w330) -> (w334:T20)  [unwired: 1 in]
        n347 = Bundle("Time"=w320, "Time"=w319, "In Minutes"=w332) -> (w336:T20)  [unwired: 1 in]
        n348 = Build Array(w336, w335, w334) -> (w333:T21)
        n349 = for {
          tunnel: "Where Shift_Id = %d" ("condition") -> [w666]
          tunnel: "master_shift" ("table") -> [w665]
          tunnel: w333 -> [w662] mode=indexing
          tunnel: w329 -> [w661]
          i -> [w668]
          n350 = Increment(x=w668) -> (x+1=w667:i32)
          n351 = Format Into String(format string=w666, w667) -> (resulting string=w663:string, error out=w669:errorcluster)  [unwired: 2 in]
          n352 = call <vilib>:"DB Tools Update Data.vi"("condition"=w663, "data"=w662, "error in (no error)"=w669, "columns"=string[] ["SHIFT_START", "SHIFT_END", "SHIFT_TIME_IN_MIN"] ("table"), "table"=w665, "connection reference"=w661) -> ()  [unwired: 4 in, 2 out]
        }
      }
      event "Cancel Button - Archive": Value Change {
        n353 = event-data() -> ()  [unwired: 1 in, 6 out]
      }
    }
  }
  n354 = call <vilib>:"DB Tools Close Connection.vi"("error in (no error)"=w281, "connection reference"=w282) -> ("error out"=w2:errorcluster)  [unwired: 5 in]
  n355 = call <vilib>:"Simple Error Handler.vi"("error in (no error)"=w2) -> ("error out"=w4:errorcluster)  [unwired: 4 in, 4 out]
  n356 = call <vilib>:"Clear Errors.vi"("error in (no error)"=w4) -> ("error out"=w3:errorcluster)  [unwired: 5 in, 1 out]
  n357 = flat-sequence {
    tunnel: w3 -> [w745]
    tunnel: [w745] -> w1
    tunnel: [w747] -> w5
    tunnel: w1 -> [w746]
    frame #0 {
    }
    frame #1 {
      n358 = disable-structure shown="Enabled" {
        disable-tunnel: [w749 _] -> w747
        disable-tunnel: w746 -> [w748 _]
        frame Enabled {
          n359 = invoke class="VI" method="FP.Close"(error in=w748) -> (error out=w749:errorcluster)  [unwired: 2 in, 2 out]
        }
        frame Disabled {
        }
      }
    }
  }
  "error out" <- w5
